vi "Memory.Pointer.Read.Subset.In Place.vi"   [LabVIEW 2016, in "LabVIEW Memory Manager.lvlib" / "Memory.Pointer.lvclass"]
uses:
  Memory.Pointer.lvclass
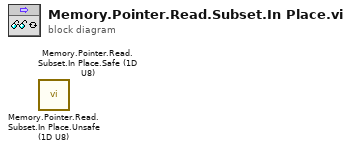
[diagram p0: block diagram]
diagram:
  n1 = call "Memory.Pointer.Read.Subset.In Place.Unsafe (1D U8).vi"() -> ()  [unwired: 8 in, 4 out]
  n2 = call "Memory.Pointer.Read.Subset.In Place.Safe (1D U8).vi"() -> ()  [unwired: 8 in, 4 out]
